vi "roi_descriptor_example_updated.vi"() -> ()   [LabVIEW 2014]
doc: "This example demonstrates how each ROI type is defined. There is a tab for each ROI type and the last tab allows you to draw an ROI and see how the ROI descriptor is changed. Please\nuse the last tab to understand the difference between Freehand ROI, Roken Line ROI, Freehand Line ROI, and Polygon ROI. As these 4 ROI types differ more in how they are drawn on\nthe IMAQ Image control and less in how they are defined in the ROI Descriptor cluster.\n\nDefinitions\n-----------------------------------\nGlobal Rectangle - is the minimum rectangle required to contain all of the contours in the ROI. With some of the vision processing algorithms, reducing the global rectangle will reduce the\namount of time an algorithm will take to process.\n\nContours - are each of the individual shapes that define the ROI. You can have multiple contours (or shapes) per ROI Descriptor.\n\nID - refers to whether the contour is the external or internal edge of an ROI. If the contour is external, all of the area inside it is considered part of the ROI. If the contour is internal then\nall of the area outside of the ROI defined lines is considered part of the ROI.\n\nType - is the shape type of the contour. \n\nCoordinates - is the coordinates that define the contour."
panel:
  in  "stop":bool
  in  "Tab Control":T1(tab)
  out "Point ROI Image Out":T2(plugin-control)
  in  "Point ROI Descriptor In":T3={"Global Rectangle"=[0, 0, 250, 250], "Contours"=[{"ID"=enum."External", "Type"=1, "Coordinates"=[50, 100]}]} {"Contours"."Type" items=["No Selection", "Point", "Line", "Rectangle", "Oval", "Polygon", "Freehand Region", "Annulus", "Unused2", "Unused3", "Broken Line", "Freehand Line", "Rotated Rectangle"]}
  out "Line ROI Image Out":T2(plugin-control)
  in  "Line ROI Descriptor In":T3={"Global Rectangle"=[0, 0, 250, 250], "Contours"=[{"ID"=enum."External", "Type"=2, "Coordinates"=[50, 100, 200, 200]}]} {"Contours"."Type" items=["No Selection", "Point", "Line", "Rectangle", "Oval", "Polygon", "Freehand Region", "Annulus", "Unused2", "Unused3", "Broken Line", "Freehand Line", "Rotated Rectangle"]}
  out "Rectangle ROI Image Out":T2(plugin-control)
  in  "Rectangle ROI Descriptor In":T3={"Global Rectangle"=[0, 0, 250, 250], "Contours"=[{"ID"=enum."External", "Type"=3, "Coordinates"=[50, 100, 200, 200]}]} {"Contours"."Type" items=["No Selection", "Point", "Line", "Rectangle", "Oval", "Polygon", "Freehand Region", "Annulus", "Unused2", "Unused3", "Broken Line", "Freehand Line", "Rotated Rectangle"]}
  out "Oval ROI Image Out":T2(plugin-control)
  in  "Oval ROI Descriptor In":T3={"Global Rectangle"=[0, 0, 250, 250], "Contours"=[{"ID"=enum."External", "Type"=4, "Coordinates"=[50, 100, 200, 200]}]} {"Contours"."Type" items=["No Selection", "Point", "Line", "Rectangle", "Oval", "Polygon", "Freehand Region", "Annulus", "Unused2", "Unused3", "Broken Line", "Freehand Line", "Rotated Rectangle"]}
  out "Polygon ROI Image Out":T2(plugin-control)
  in  "Polygon ROI Descriptor In":T3={"Global Rectangle"=[0, 0, 250, 250], "Contours"=[{"ID"=enum."External", "Type"=5, "Coordinates"=[10, 10, 200, 15, 190, 150, 125, 100]}]} {"Contours"."Type" items=["No Selection", "Point", "Line", "Rectangle", "Oval", "Polygon", "Freehand Region", "Annulus", "Unused2", "Unused3", "Broken Line", "Freehand Line", "Rotated Rectangle"]}
  out "Freehand ROI Image Out":T2(plugin-control)
  in  "Freehand ROI Descriptor In":T3={"Global Rectangle"=[0, 0, 250, 250], "Contours"=[{"ID"=enum."External", "Type"=6, "Coordinates"=[10, 10, 50, 10, 20, 25, 10, 10]}]} {"Contours"."Type" items=["No Selection", "Point", "Line", "Rectangle", "Oval", "Polygon", "Freehand Region", "Annulus", "Unused2", "Unused3", "Broken Line", "Freehand Line", "Rotated Rectangle"]}
  out "Annulus ROI Image Out":T2(plugin-control)
  in  "Annulus ROI Descriptor In":T3={"Global Rectangle"=[0, 0, 250, 250], "Contours"=[{"ID"=enum."External", "Type"=7, "Coordinates"=[125, 125, 50, 100, 100000, 300000]}]} {"Contours"."Type" items=["No Selection", "Point", "Line", "Rectangle", "Oval", "Polygon", "Freehand Region", "Annulus", "Unused2", "Unused3", "Broken Line", "Freehand Line", "Rotated Rectangle"]}
  out "Broken Line ROI Image Out":T2(plugin-control)
  in  "Broken Line ROI Descriptor In":T3={"Global Rectangle"=[0, 0, 250, 250], "Contours"=[{"ID"=enum."External", "Type"=10, "Coordinates"=[10, 10, 200, 15, 190, 150, 125, 100]}]} {"Contours"."Type" items=["No Selection", "Point", "Line", "Rectangle", "Oval", "Polygon", "Freehand Region", "Annulus", "Unused2", "Unused3", "Broken Line", "Freehand Line", "Rotated Rectangle"]}
  out "Freehand Line ROI Image Out":T2(plugin-control)
  in  "Freehand Line ROI Descriptor In":T3={"Global Rectangle"=[0, 0, 250, 250], "Contours"=[{"ID"=enum."External", "Type"=11, "Coordinates"=[10, 10, 50, 10, 20, 25]}]} {"Contours"."Type" items=["No Selection", "Point", "Line", "Rectangle", "Oval", "Polygon", "Freehand Region", "Annulus", "Unused2", "Unused3", "Broken Line", "Freehand Line", "Rotated Rectangle"]}
  out "Rotated Rectangle ROI Image Out":T2(plugin-control)
  in  "Rotated Rectangle ROI Descriptor In":T3={"Global Rectangle"=[0, 0, 250, 250], "Contours"=[{"ID"=enum."External", "Type"=12, "Coordinates"=[50, 100, 200, 200, 56555]}]} {"Contours"."Type" items=["No Selection", "Point", "Line", "Rectangle", "Oval", "Polygon", "Freehand Region", "Annulus", "Unused2", "Unused3", "Broken Line", "Freehand Line", "Rotated Rectangle"]}
  out "ROI Descriptor Out":T3={"Global Rectangle"=[24, 100, 149, 196], "Contours"=[{"ID"=enum."External", "Type"=5, "Coordinates"=[24, 143, 108, 100, 148, 147, 83, 195, 24, 143]}]} {"Contours"."Type" items=["No Selection", "Point", "Line", "Rectangle", "Oval", "Polygon", "Freehand Region", "Annulus", "Unused2", "Unused3", "Broken Line", "Freehand Line", "Rotated Rectangle"]}
  out "ROI Image In":T2(plugin-control)
  # "Overview: This example gives an in-depth explanation of Vision ROI descriptors. It details how each ROI type descriptor is represented and defined in LabVIEW.\nRequirements: LabVIEW Full Development System 2014 and Vision Development Module 2014 and later\nInstructions:\n1. Run VI \n2. Go through the tabs to learn about the different ROI types. Observe the Descriptor Cluster for the ROI that is already drawn in each IMAQ Image Control.\n3. Go to the last tab \"Draw ROI\" and draw a ROI on the IMAQ Image Control. Single left click creates a point and double left click completes the ROI."
  # "Point ROI\n\nThe first element in the Coordinates array defines\nthe X and the second element defines Y.\n\nOn the right we have created a point at X = 50 and\nY = 100."
  # "Line ROI\n\nCoordinates Array\n---------------------------------\nElement 0: X1\nElement 1: Y1\nElement 2: X2\nElement 3: Y2\n\nOn the right we have created a line at X = 50 and\nY = 100.  We have created another point at\nX = 200 and Y = 200.  The line is drawn between\nthe two points."
  # "Rectangle ROI\n\nCoordinates Array\n---------------------------------\nElement 0: X Left Boundary\nElement 1: Y Top Boundary\nElement 2: X Right Boundary\nElement 3: Y Bottom Boundary\n\nOn the right we have created a rectangle defined\nby four boundaries.  X1 = 50, Y1 = 100, X2 = 200,\nand Y2 = 200."
  # "Oval ROI\n\nCoordinates Array\n---------------------------------\nElement 0: X Left Boundary\nElement 1: Y Top Boundary\nElement 2: X Right Boundary\nElement 3: Y Bottom Boundary\n\nOn the right we have created an oval defined\nby four boundaries.  X1 = 50, Y1 = 100, X2 = 200,\nand Y2 = 200.  Notice how similar this is to the\nrectangle ROI."
  # "Polygon ROI\n\nCoordinates Array\n---------------------------------\nElement 0: X1\nElement 1: Y1\nElement 2: X2\nElement 3: Y2\nElement 4: X3\nElement 5: Y4\n.\n.\n.\n\nThe freehand, polygon, broken line, and freehand\nline ROIs are all defined the same way.  By manipulating\nthe Coordinate array you will not be able to tell the\ndifference between the 4 types of ROIs.  There difference\nlies in how the IMAQ Image control creates these ROIs.\n\nPolygon Attribute 1:  Polygon is created by placing points on\nthe IMAQ Image control and double clicking the mouse when\nyou are done (this is in contrast to Freehand in which you\ndraw the ROI like you were usign a Pen).\n\nPolygon Attribute 2:  When finsihed drawing the last\npoint is connected to the first point (this is in contrast to\nBroken Line).\n\nPolygon Attribute 3:  After displaying the ROI the user can\nmove individual points around."
  # "Freehand ROI\n\nCoordinates Array\n---------------------------------\nElement 0: X1\nElement 1: Y1\nElement 2: X2\nElement 3: Y2\nElement 4: X3\nElement 5: Y4\n.\n.\n.\n\nThe freehand, polygon, broken line, and freehand\nline ROIs are all defined the same way.  By manipulating\nthe Coordinate array you will not be able to tell the\ndifference between the 4 types of ROIs.  There difference\nlies in how the IMAQ Image control creates these ROIs.\n\nFreehand Attribute 1:  Pen type drawing when using IMAQ\nImage control to draw (this is in contrast to Polygon and\nBroken Line).\n\nFreehand Attribute 2:  When finsihed drawing the last\npoint is connected to the first point (this is in contrast to\nFreehand Line)."
  # "Annulus ROI\n\nCoordinates Array\n---------------------------------\nElement 0: X value defining center of Annulus\nElement 1: Y value defining center of Annulus\nElement 2: Radius of Inner Circle\nElement 3: Radius of Outer Circle\nElement 4: Angle 1\nElement 5: Angle 2\n\nAngles\n-----------\n1.  Angles are defined with 3 digits of precision\nwithout a period to indicate which numbers are\ndecimals.\n\n2.  Angles are defined in degrees.\n\nFor example:\n120 degrees is 120000\n94 degrees is 94000\n122.12 degrees is 122120\n1.221 degrees is 1221"
  # "Broken Line ROI\n\nCoordinates Array\n---------------------------------\nElement 0: X1\nElement 1: Y1\nElement 2: X2\nElement 3: Y2\nElement 4: X3\nElement 5: Y4\n.\n.\n.\n\nThe freehand, polygon, broken line, and freehand\nline ROIs are all defined the same way.  By manipulating\nthe Coordinate array you will not be able to tell the\ndifference between the 4 types of ROIs.  There difference\nlies in how the IMAQ Image control creates these ROIs.\n\nBroken Line Attribute 1:  Broken Line is created by placing\npoints on the IMAQ Image control and double clicking the\nmouse when you are done (this is in contrast to Freehand\nin which you draw the ROI like you were usign a Pen).\n\nBroken Line Attribute 2:  When finsihed drawing the last\npoint is not connected to the first point (this is in contrast to\nPolygon).\n\nBroken Line Attribute 3:  After displaying the ROI the user can\nmove individual points around."
  # "Freehand Line ROI\n\nCoordinates Array\n---------------------------------\nElement 0: X1\nElement 1: Y1\nElement 2: X2\nElement 3: Y2\nElement 4: X3\nElement 5: Y4\n.\n.\n.\n\nThe freehand, polygon, broken line, and freehand\nline ROIs are all defined the same way.  By manipulating\nthe Coordinate array you will not be able to tell the\ndifference between the 4 types of ROIs.  There difference\nlies in how the IMAQ Image control creates these ROIs.\n\nFreehand Line Attribute 1:  Pen type drawing when using\nIMAQ Image control to draw (this is in contrast to Polygon\nand Broken Line).\n\nFreehand Line Attribute 2:  When finsihed drawing the\nlast point is not connected to the first point (this is in\ncontrast to Freehand)."
  # "Enter ROI by Hand"
  # "Rotated Rectangle ROI\n\nCoordinates Array\n---------------------------------\nElement 0: X Left Boundary\nElement 1: Y Top Boundary\nElement 2: X Right Boundary\nElement 3: Y Bottom Boundary\nElement 4: Angle of Rotation\n\nVery similar to Rectangle ROI except that\nyou can define an angle.\n\nAngles\n-----------\n1.  Angles are defined with 3 digits of precision\nwithout a period to indicate which numbers are\ndecimals.\n\n2.  Angles are defined in degrees.\n\nFor example:\n120 degrees is 120000\n94 degrees is 94000\n122.12 degrees is 122120\n1.221 degrees is 1221"
  # "Draw the ROI on the IMAGE Control"
  # "Draw the ROI\n\nPlease take the time to draw a Polygon,\nFreehand, Broken Line, and Freehand\nLine ROI and see how they differ\nwhen drawing these ROIs.  This\nwill show why they are different\ntypes in the ROI Descriptor.\nOne click creates a point. Double click finishes\nthe ROI."
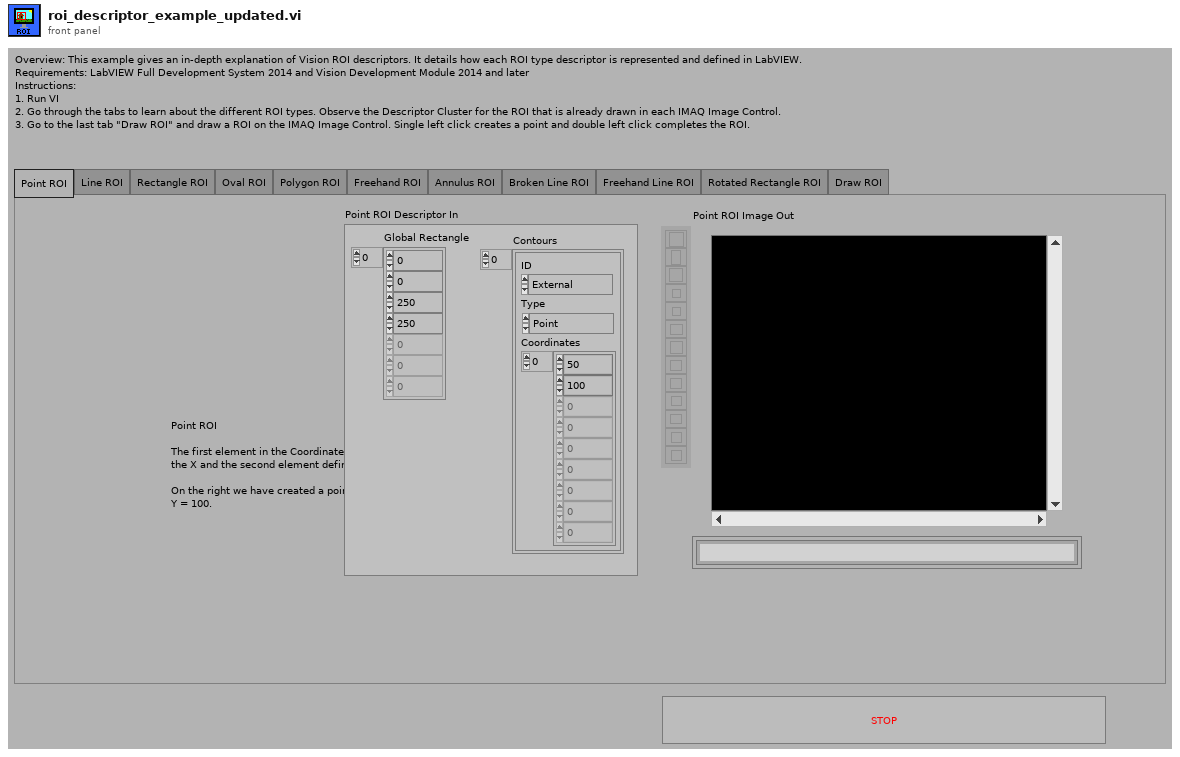
[diagram p1: front panel]
types:
  T1 = enum32{"Point ROI", "Line ROI", "Rectangle ROI", "Oval ROI", "Polygon ROI", "Freehand ROI", "Annulus ROI", "Broken Line ROI", "Freehand Line ROI", "Rotated Rectangle ROI", "Draw ROI"}
  T2 = typedef "IMAQ Image.ctl" = refnum<image>
  T3 = typedef "ROI Descriptor" = cluster{"Global Rectangle":i32[], "Contours":cluster{"ID":enum32{"External", "Internal"}, "Type":u32, "Coordinates":i32[]}[]}
  T4 = cluster{"Global Rectangle":i32[], "Contours":cluster{"Contour Type":u32, "ROI Type":u32, "Points":i32[]}[]}
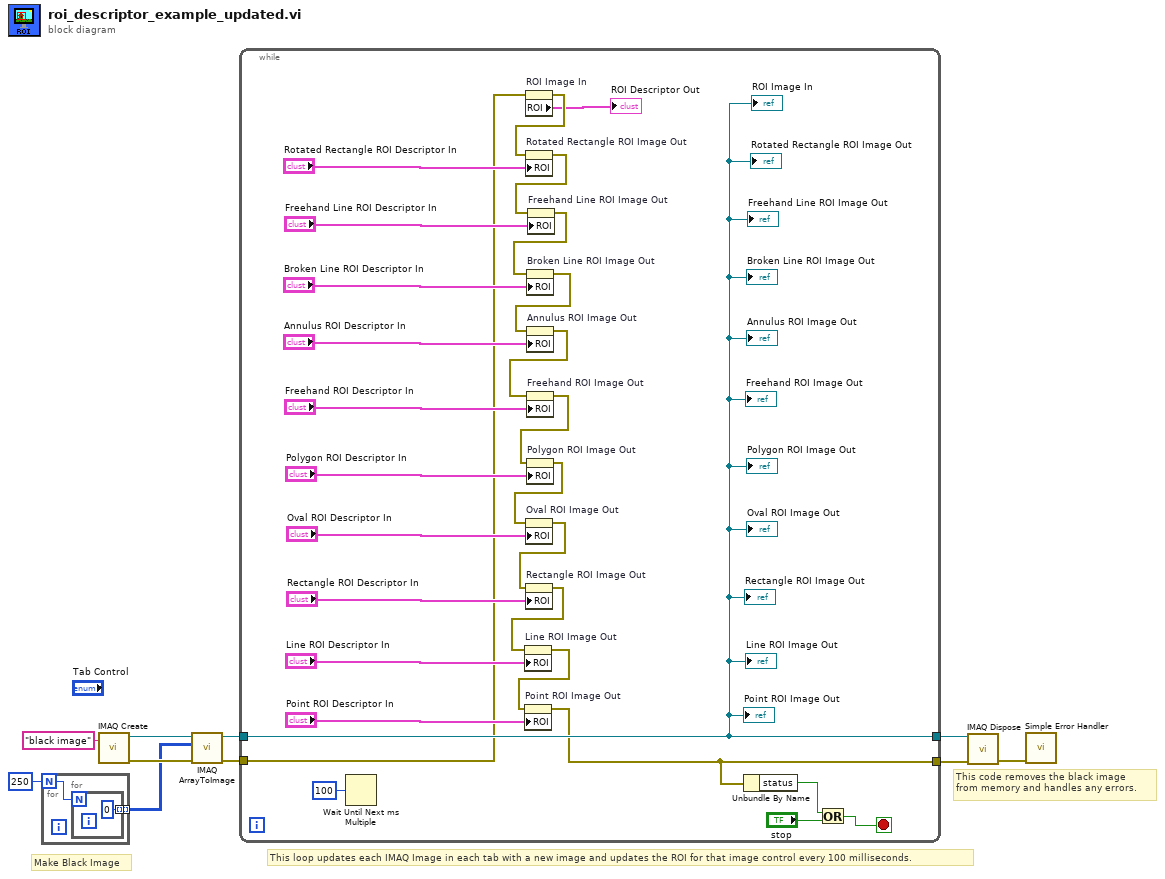
[diagram p0: block diagram]
diagram:
  # "This code removes the black image\nfrom memory and handles any errors."
  # "This loop updates each IMAQ Image in each tab with a new image and updates the ROI for that image control every 100 milliseconds."
  # "Make Black Image"
  n1 = for {
    N: 250 -> [w11]
    tunnel: [w12] -> w7 mode=indexing
    n2 = for {
      N: w11 -> [_]
      tunnel: [u8 0] -> w12 mode=indexing
    }
  }
  n3 = call "IMAQ Create"("Image Name"="black image") -> ("New Image"=w9:T2, "error out"=w8:errorcluster)  [unwired: 4 in]
  n4 = call "IMAQ ArrayToImage"("error in (no error)"=w8, "Image Pixels (U8)"=w7, "Image"=w9) -> ("error out"=w5:errorcluster, "Image Out"=w6:T2)  [unwired: 7 in]
  n5 = while {
    tunnel: w6 -> [w18]
    tunnel: w5 -> [w17]
    tunnel: [w14] -> w4
    tunnel: [w18] -> w3
    stop <- w39 stop-if-true
    n6 = Wait Until Next ms Multiple(millisecond multiple=u32 100) -> ()  [unwired: 1 out]
    n7 = property on="ROI Image In" class="ImageControl"(error in=w17) -> (error out=w16:errorcluster, "ROI"=→"ROI Descriptor Out":T4)  [unwired: 1 in, 1 out]
    n8 = property on="Rotated Rectangle ROI Image Out" class="ImageControl"(error in=w16, "ROI"="Rotated Rectangle ROI Descriptor In") -> (error out=w21:errorcluster)  [unwired: 1 in, 1 out]
    n9 = property on="Freehand Line ROI Image Out" class="ImageControl"(error in=w21, "ROI"="Freehand Line ROI Descriptor In") -> (error out=w23:errorcluster)  [unwired: 1 in, 1 out]
    n10 = property on="Broken Line ROI Image Out" class="ImageControl"(error in=w23, "ROI"="Broken Line ROI Descriptor In") -> (error out=w25:errorcluster)  [unwired: 1 in, 1 out]
    n11 = property on="Annulus ROI Image Out" class="ImageControl"(error in=w25, "ROI"="Annulus ROI Descriptor In") -> (error out=w27:errorcluster)  [unwired: 1 in, 1 out]
    n12 = property on="Freehand ROI Image Out" class="ImageControl"(error in=w27, "ROI"="Freehand ROI Descriptor In") -> (error out=w29:errorcluster)  [unwired: 1 in, 1 out]
    n13 = property on="Polygon ROI Image Out" class="ImageControl"(error in=w29, "ROI"="Polygon ROI Descriptor In") -> (error out=w31:errorcluster)  [unwired: 1 in, 1 out]
    n14 = property on="Oval ROI Image Out" class="ImageControl"(error in=w31, "ROI"="Oval ROI Descriptor In") -> (error out=w33:errorcluster)  [unwired: 1 in, 1 out]
    n15 = property on="Rectangle ROI Image Out" class="ImageControl"(error in=w33, "ROI"="Rectangle ROI Descriptor In") -> (error out=w34:errorcluster)  [unwired: 1 in, 1 out]
    n16 = property on="Line ROI Image Out" class="ImageControl"(error in=w34, "ROI"="Line ROI Descriptor In") -> (error out=w19:errorcluster)  [unwired: 1 in, 1 out]
    n17 = property on="Point ROI Image Out" class="ImageControl"(error in=w19, "ROI"="Point ROI Descriptor In") -> (error out=w14:errorcluster)  [unwired: 1 in, 1 out]
    n18 = Unbundle By Name(w14) -> ("status"=w38:bool)
    n19 = Or(x=w38, y="stop") -> (x .or. y?=w39:bool)
    "Point ROI Image Out" <- w18
    "Line ROI Image Out" <- w18
    "Rectangle ROI Image Out" <- w18
    "Oval ROI Image Out" <- w18
    "Polygon ROI Image Out" <- w18
    "Freehand ROI Image Out" <- w18
    "Annulus ROI Image Out" <- w18
    "Broken Line ROI Image Out" <- w18
    "Freehand Line ROI Image Out" <- w18
    "Rotated Rectangle ROI Image Out" <- w18
    "ROI Image In" <- w18
  }
  n20 = call "IMAQ Dispose"("Image"=w3, "error in (no error)"=w4) -> ("error out"=w1:errorcluster)  [unwired: 4 in]
  n21 = call <vilib>:"Simple Error Handler.vi"("error in (no error)"=w1) -> ()  [unwired: 4 in, 5 out]
